vi "gxml_UnflattenAndScanItem.vi"(7 "Disable Parse?":bool, 8 "error in":errorcluster, 9 "Offset In":i32, 10 "FlattenedData":string, 11 "variant":variant) -> (0 "error out":errorcluster, 1 "Offset Out":i32, 3 "Data Info":T1, 5 "Enum?":bool)   [LabVIEW 2011, in "Third Party VIs.lvlib" / "GXML.lvlib"]
uses:
  GXML.lvlib
  <vilib>/Utility/VariantDataType/VariantType.lvlib
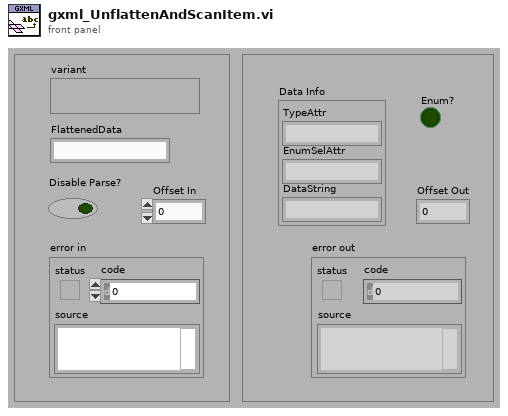
[diagram p1: front panel]
types:
  T1 = cluster{"TypeAttr":string, "EnumSelAttr":string, "DataString":string}
  T2 = typedef "VariantType.lvlib/Type.ctl" = enum8{"Invalid Type", "Void", "I8", "I16", "I32", "I64", "U8", "U16", "U32", "U64", "Single Float", "Double Float", "Extended Float", "Single Complex", "Double Complex", "Extended Complex", "Enum U8", "Enum U16", "Enum U32", "Enum U64", "Single Float With Unit", "Double Float With Unit", "Extended Float With Unit", "Single Complex with Unit", "Double Complex with Unit", "Extended Complex with Unit", "Boolean", "String", "Path", "Picture", "Tag", "Array", "Cluster", "Variant", "LV Variant", "Waveform", "Timestamp", "Digital Waveform", "Digital Data", "ExpressData", "Refnum", "External Data", "VI", "Poly VI", "LabVIEW Class Instance", "Fixed Point"}
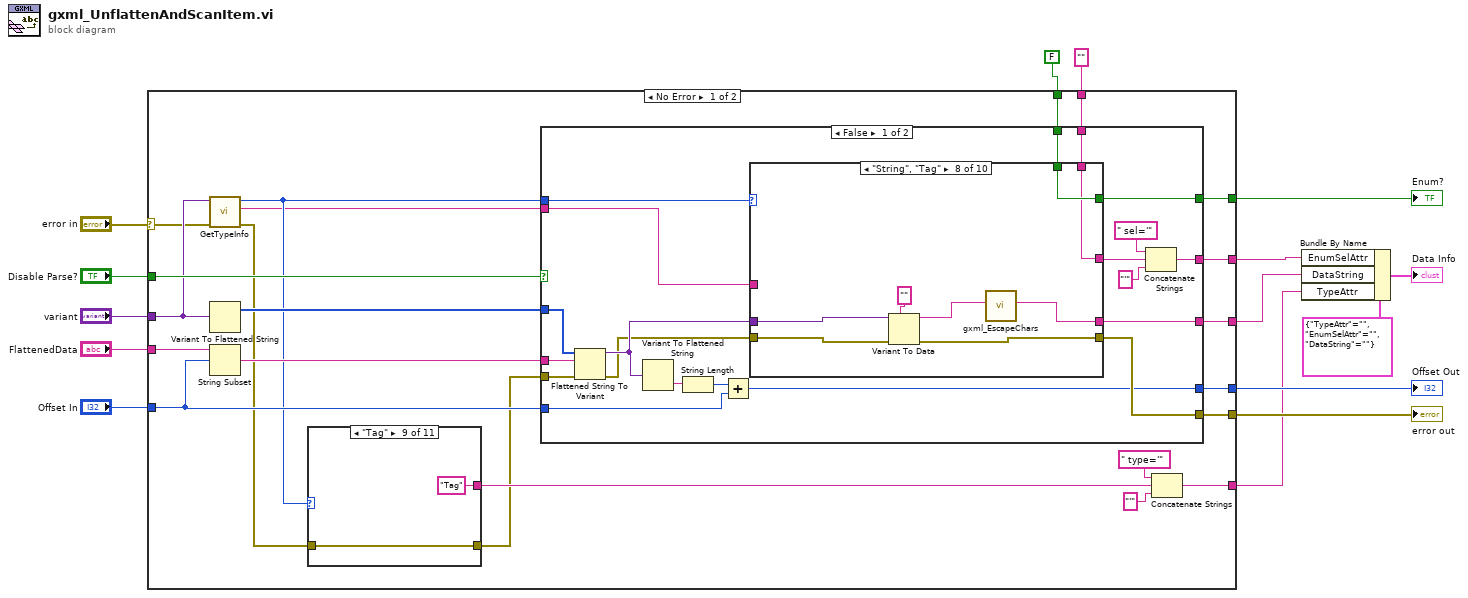
[diagram p0: block diagram]
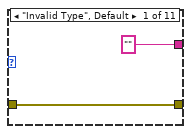
[diagram p2: hidden frame]
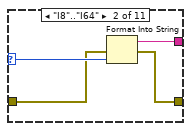
[diagram p3: hidden frame]
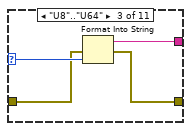
[diagram p4: hidden frame]
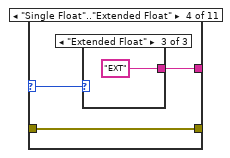
[diagram p5: hidden frame]
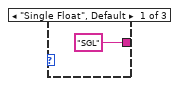
[diagram p6: hidden frame]
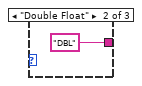
[diagram p7: hidden frame]
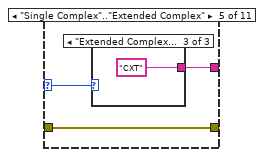
[diagram p8: hidden frame]
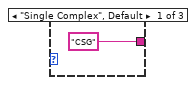
[diagram p9: hidden frame]
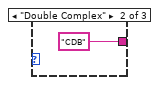
[diagram p10: hidden frame]
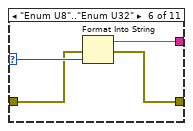
[diagram p11: hidden frame]
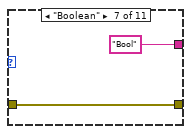
[diagram p12: hidden frame]
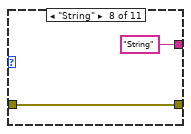
[diagram p13: hidden frame]
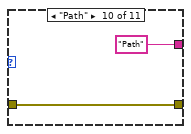
[diagram p14: hidden frame]
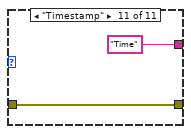
[diagram p15: hidden frame]
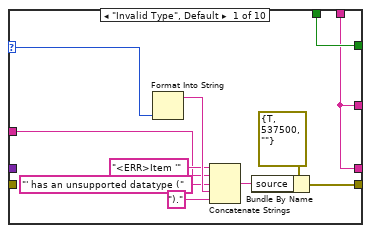
[diagram p16: hidden frame]
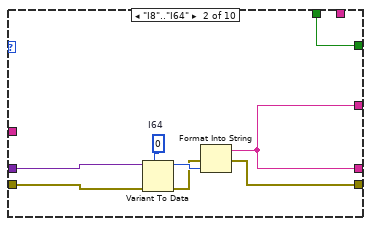
[diagram p17: hidden frame]
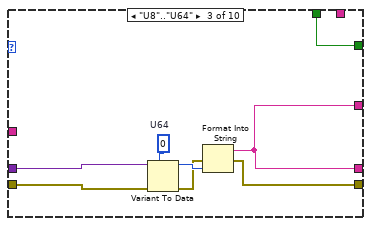
[diagram p18: hidden frame]
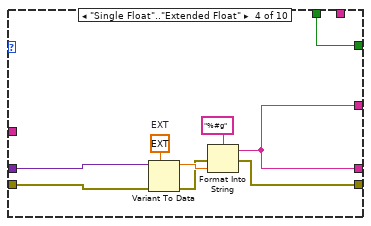
[diagram p19: hidden frame]
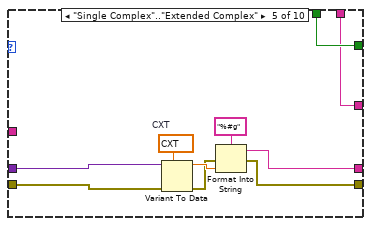
[diagram p20: hidden frame]
diagram:
  n1 = case shown="No Error" "error in" {
    selector: "error in" -> [w26 w188]
    tunnel: [w37 w188] -> w15
    tunnel: "Offset In" -> [w36 w189]
    tunnel: [w35 w189] -> w13
    tunnel: [w34 w186] -> w3
    tunnel: [w33 w187] -> w12
    tunnel: [w32 w186] -> w4
    tunnel: "Disable Parse?" -> [w30 _]
    tunnel: "FlattenedData" -> [w28 _]
    tunnel: "variant" -> [w27 _]
    tunnel: "" -> [w25 w186]
    tunnel: FALSE -> [w24 w187]
    tunnel: [w20 w186] -> w1
    frame No Error {
      n2 = call <vilib>:"GetTypeInfo.vi"("error in (no error)"=w26, "Variant"=w27) -> ("error out"=w18:errorcluster, "Name"=w16:string, "Type Enum"=w19:T2)  [unwired: 5 in, 2 out]
      n3 = Variant To Flattened String(Variant=w27) -> (1:w29:i16[])  [unwired: 1 out]
      n4 = String Subset(string=w28, offset (0)=w36) -> (substring=w31:string)  [unwired: 1 in]
      n5 = case shown="\"Tag\"" w19 {
        selector: w19 -> [_ w43 w47 w50 w56 w63 _ _ _ _ _]
        tunnel: ["" w42 w46 w49 w55 w62 "Bool" "String" "Tag" "Path" "Time"] -> w21
        tunnel: w18 -> [w38 w41 w45 w48 w54 w61 w64 w66 w69 w70 w72]
        tunnel: [w38 w40 w44 w48 w54 w60 w64 w66 w69 w70 w72] -> w17
        frame "Invalid Type", Default {
        }
        frame "I8".."I64" {
          n6 = Format Into String(error in=w41, w43) -> (resulting string=w42:string, error out=w40:errorcluster)  [unwired: 2 in]
        }
        frame "U8".."U64" {
          n7 = Format Into String(error in=w45, w47) -> (resulting string=w46:string, error out=w44:errorcluster)  [unwired: 2 in]
        }
        frame "Single Float".."Extended Float" {
          n8 = case shown="\"Extended Float\"" w50 {
            tunnel: ["SGL" "DBL" "EXT"] -> w49
            frame "Single Float", Default {
            }
            frame "Double Float" {
            }
            frame "Extended Float" {
            }
          }
        }
        frame "Single Complex".."Extended Complex" {
          n9 = case shown="\"Extended Complex\"" w56 {
            tunnel: ["CSG" "CDB" "CXT"] -> w55
            frame "Single Complex", Default {
            }
            frame "Double Complex" {
            }
            frame "Extended Complex" {
            }
          }
        }
        frame "Enum U8".."Enum U32" {
          n10 = Format Into String(error in=w61, w63) -> (resulting string=w62:string, error out=w60:errorcluster)  [unwired: 2 in]
        }
        frame "Boolean" {
        }
        frame "String" {
        }
        frame "Tag" {
        }
        frame "Path" {
        }
        frame "Timestamp" {
        }
      }
      n11 = case shown="False" w30 {
        tunnel: w17 -> [w93 w184]
        tunnel: [w92 w184] -> w37
        tunnel: w36 -> [w91 w185]
        tunnel: [w90 w185] -> w35
        tunnel: [w89 w182] -> w34
        tunnel: w29 -> [w88 _]
        tunnel: [w87 w183] -> w33
        tunnel: [w86 w182] -> w32
        tunnel: w31 -> [w78 _]
        tunnel: w19 -> [w77 _]
        tunnel: w25 -> [w76 w182]
        tunnel: w24 -> [w75 w183]
        tunnel: w16 -> [w74 _]
        frame False {
          n12 = Flattened String To Variant(4:w93, 6:w78, 7:w88) -> (0:w82:errorcluster, 3:w83:variant)
          n13 = Variant To Flattened String(Variant=w83) -> (data string=w85:string)  [unwired: 1 out]
          n14 = String Length(string=w85) -> (length=w84:i32)
          n15 = Add(x=w84, y=w91) -> (x+y=w90:i32)
          n16 = case shown="\"String\", \"Tag\"" w77 {
            selector: w77 -> [w103 _ _ _ _ _ _ _ _ _]
            tunnel: w83 -> [_ w112 w119 w128 w137 w144 w154 w162 w170 w176]
            tunnel: w82 -> [_ w105 w113 w127 w136 w140 w153 w157 w169 w175]
            tunnel: [w98 w107 w115 w122 w135 w142 w150 w155 w163 w174] -> w89
            tunnel: [w104 w108 w116 w124 w133 w143 w148 w160 w165 w173] -> w92
            tunnel: [w98 w107 w115 w122 w130 w141 w146 w158 w167 w180] -> w80
            tunnel: [w99 w106 w114 w121 w131 TRUE w147 w159 w168 w181] -> w87
            tunnel: w75 -> [w99 w106 w114 w121 w131 _ w147 w159 w168 w181]
            tunnel: w76 -> [w98 _ _ _ w130 _ w146 w158 w167 w180]
            tunnel: w74 -> [w96 _ _ _ _ _ _ _ _ _]
            frame "Invalid Type", Default {
              n17 = Format Into String(w103) -> (resulting string=w100:string)  [unwired: 3 in, 1 out]
              n18 = Concatenate Strings("<ERR>Item '" ("Format String"), w96, "' has an unsupported datatype (" ("Format String"), w100, ")." ("string")) -> (w101:string)
              n19 = Bundle By Name(cluster=errorcluster {"status"=TRUE, "code"=537500, "source"=""} ("error in"), "source"=w101) -> (w104:errorcluster)
            }
            frame "I8".."I64" {
              w111 = i64 0  # I64
              n20 = Variant To Data(error in=w105, type=w111, Variant=w112) -> (data=w110:i64, error out=w109:errorcluster)
              n21 = Format Into String(error in=w109, w110) -> (resulting string=w107:string, error out=w108:errorcluster)  [unwired: 2 in]
            }
            frame "U8".."U64" {
              w120 = u64 0  # U64
              n22 = Variant To Data(error in=w113, type=w120, Variant=w119) -> (data=w118:u64, error out=w117:errorcluster)
              n23 = Format Into String(error in=w117, w118) -> (resulting string=w115:string, error out=w116:errorcluster)  [unwired: 2 in]
            }
            frame "Single Float".."Extended Float" {
              w129 = ext 0.0  # EXT
              n24 = Variant To Data(error in=w127, type=w129, Variant=w128) -> (data=w126:ext, error out=w125:errorcluster)
              n25 = Format Into String(format string="%#g", error in=w125, w126) -> (resulting string=w122:string, error out=w124:errorcluster)  [unwired: 1 in]
            }
            frame "Single Complex".."Extended Complex" {
              w139 = cxt 0.0+0.0i  # CXT
              n26 = Variant To Data(error in=w136, type=w139, Variant=w137) -> (data=w138:cxt, error out=w134:errorcluster)
              n27 = Format Into String(format string="%#g", error in=w134, w138) -> (resulting string=w135:string, error out=w133:errorcluster)  [unwired: 1 in]
            }
            frame "Enum U8".."Enum U32" {
              n28 = call "gxml_GetEnumTxt.vi"("error in"=w140, "Enum"=w144) -> ("error out"=w143:errorcluster, "String Value"=w141:string, "SelectionNum"=w142:string)  [unwired: 7 in]
            }
            frame "Boolean" {
              n29 = Variant To Data(error in=w153, type=FALSE, Variant=w154) -> (data=w151:bool, error out=w149:errorcluster)
              n30 = Format Into String(error in=w149, w151) -> (resulting string=w150:string, error out=w148:errorcluster)  [unwired: 2 in]
            }
            frame "String", "Tag" {
              n31 = Variant To Data(error in=w157, type="", Variant=w162) -> (data=w156:string, error out=w160:errorcluster)
              n32 = call "gxml_EscapeChars.vi"("XML In"=w156) -> ("XML Out"=w155:string)  [unwired: 10 in]
            }
            frame "Path" {
              n33 = Variant To Data(error in=w169, type=path "", Variant=w170) -> (data=w166:path, error out=w165:errorcluster)
              n34 = Path To String(path=w166) -> (string=w164:string)
              n35 = call "gxml_EscapeChars.vi"("XML In"=w164) -> ("XML Out"=w163:string)  [unwired: 10 in]
            }
            frame "Timestamp" {
              n36 = Variant To Data(error in=w175, type=timestamp(0 s since 1904-01-01) ("time stamp"), Variant=w176) -> (data=w178:timestamp, error out=w177:errorcluster)
              n37 = Format Into String(format string="%<%H:%M:%S %x>T", error in=w177, w178) -> (resulting string=w174:string, error out=w173:errorcluster)  [unwired: 1 in]
            }
          }
          n38 = Concatenate Strings(" sel='", w80, "'" ("string")) -> (w86:string)
        }
        frame True {
        }
      }
      n39 = Concatenate Strings(" type='" ("string"), w21, "'" ("string")) -> (w20:string)
    }
    frame Error {
    }
  }
  "error out" <- w15
  "Offset Out" <- w13
  "Enum?" <- w12
  n40 = Bundle By Name(cluster=T1 {"TypeAttr"="", "EnumSelAttr"="", "DataString"=""}, "EnumSelAttr"=w4, "DataString"=w3, "TypeAttr"=w1) -> (→"Data Info":T1)
